vi "Recurse.vi"(6 "Teller":refnum<class "Teller.lvclass">, 7 "Actor in":refnum<class "Actor.lvclass">, 8 "Error in":errorcluster, 9 "Error":errorcluster, 10 "Actor":refnum<class "Actor.lvclass">) -> (0 "Error out":errorcluster, 5 "Actor out":refnum<class "Actor.lvclass">)   [LabVIEW 2020, in "jettl.lvlib" / "Stopped jettl Msg.lvlib" / "Stopped.lvlib"]
uses:
  Stopped.lvlib
  jettl.lvlib
  Stopped Msg Output/Stopped Msg Output.lvlib
  Init Msg.vi
  Actor/Actor.lvclass
  Teller/Teller.lvclass
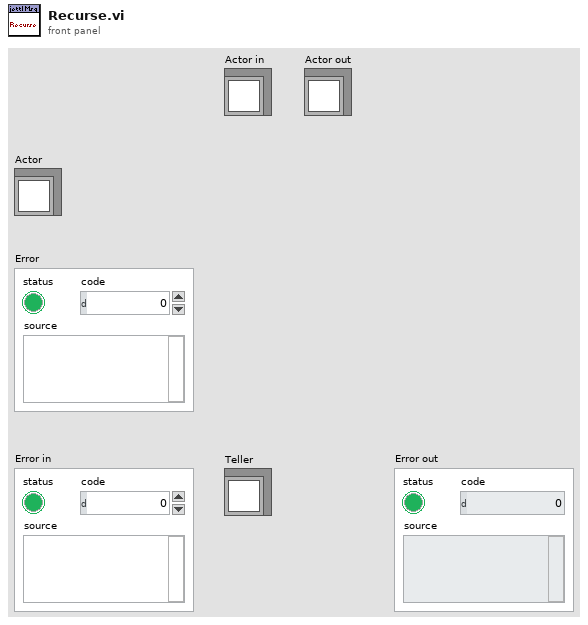
[diagram p1: front panel]
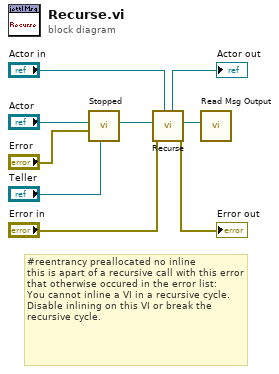
[diagram p0: block diagram]
diagram:
  # "#reentrancy preallocated no inline\nthis is apart of a recursive call with this error that otherwise occured in the error list:\nYou cannot inline a VI in a recursive cycle. Disable inlining on this VI or break the recursive cycle."
  n1 = call-poly "Stopped.vi"("Teller"="Teller", "Error"="Error", "Actor"="Actor") -> ("Msg"=w4:refnum<class "Msg.lvclass">)  [unwired: 8 in]
  n2 = call "Recurse.vi"("Actor in"="Actor in", "Error in"="Error in", "Msg"=w4) -> ("Error out"=→"Error out":errorcluster, "Msg Output"=w5:refnum<class "Msg Output.lvclass">, "Actor out"=→"Actor out":refnum<class "Actor.lvclass">)  [unwired: 6 in]
  n3 = call "Read Msg Output.vi"("Msg Output"=w5) -> ()  [unwired: 11 in]
